vi "Read iaa.vi"(8 "error in (no error)":errorcluster, 11 "RotOffset in":refnum<class "RotOffset.lvclass">) -> (0 "error out":errorcluster, 2 "iaa":dbl[unit] min=0.0 max=6.283185307179586, 3 "RotOffset out":refnum<class "RotOffset.lvclass">)   [LabVIEW 2022 SP3, in "TCSDataDefinitions.lvlib" / "TCSCommand.lvlib" / "OffsetCommands.lvlib" / "RotOffset.lvclass"]
uses:
  RotOffset.lvclass
  RotOffset.lvclass/RotOffset.ctl
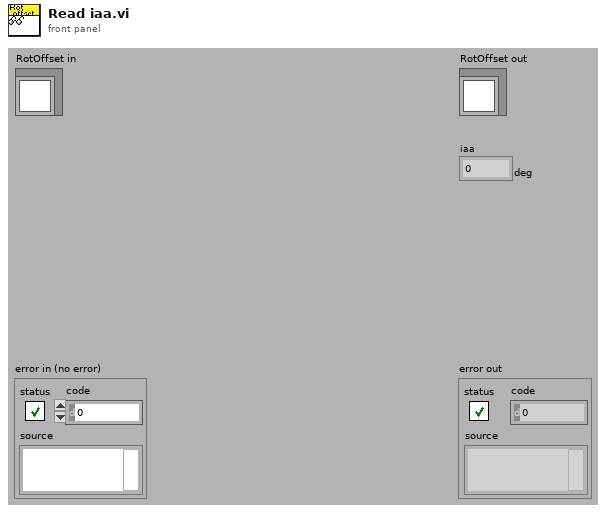
[diagram p1: front panel]
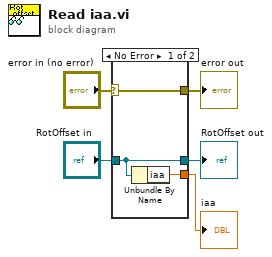
[diagram p0: block diagram]
diagram:
  n1 = case shown="No Error" "error in (no error)" {
    selector: "error in (no error)" -> [w8 w9]
    tunnel: [w8 w9] -> w4
    tunnel: [w7 w10] -> w2
    tunnel: "RotOffset in" -> [w7 w10]
    tunnel: [w6 _] -> w1
    frame No Error {
      n2 = Unbundle By Name(w7) -> ("iaa"=w6:dbl[unit])
    }
    frame Error {
    }
  }
  "error out" <- w4
  "RotOffset out" <- w2
  "iaa" <- w1
